vi "Add Result.vi"(8 "error in (no error)":errorcluster, 10 "Result":refnum<class "Result.lvclass">, 11 "Results in":refnum<class "Results.lvclass">) -> (0 "error out":errorcluster, 3 "Results out":refnum<class "Results.lvclass">)   [LabVIEW 2018, in "InfluxDB Client.lvlib" / "Results.lvclass"]
uses:
  Results.lvclass
  Result/Result.lvclass
  Results.lvclass/Results.ctl
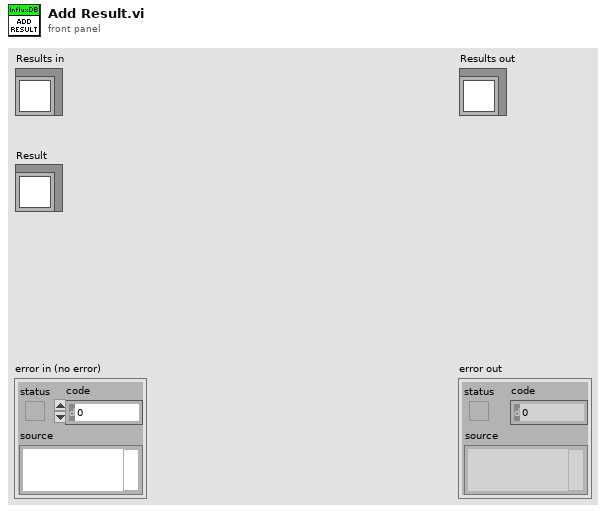
[diagram p1: front panel]
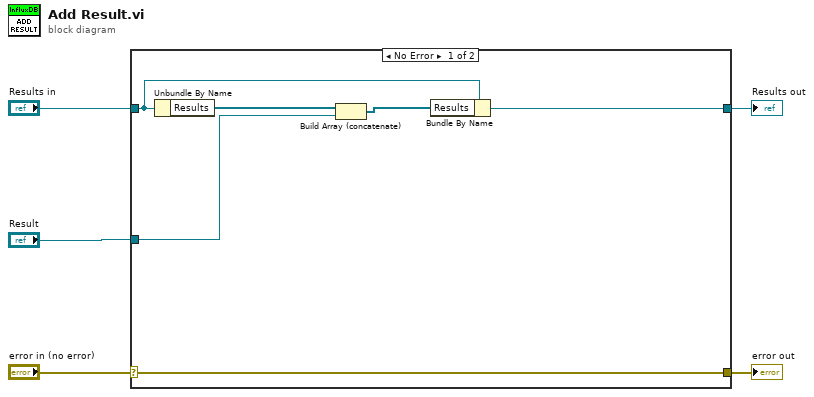
[diagram p0: block diagram]
diagram:
  n1 = case shown="No Error" "error in (no error)" {
    selector: "error in (no error)" -> [w11 w13]
    tunnel: [w11 w13] -> w4
    tunnel: [w7 w12] -> w2
    tunnel: "Results in" -> [w8 w12]
    tunnel: "Result" -> [w10 _]
    frame No Error {
      n2 = Unbundle By Name(w8) -> ("Results"=w9:refnum<class "Result.lvclass">[])
      n3 = Build Array (concatenate)(w9, w10) -> (w6:refnum<class "Result.lvclass">[])
      n4 = Bundle By Name(cluster=w8, "Results"=w6) -> (w7:refnum<class "Results.lvclass">)
    }
    frame Error {
    }
  }
  "error out" <- w4
  "Results out" <- w2
